vi "Verify powerup.vi"(0 "Measurement Configuration":T3={"Quick Power Down"=FALSE, "Pin Name"=[], "Source Mode"=[], "Start Value"=[], "Target Value"=[], "Compliance Limit"=[], "Sense Mode"=[], "Default Ramp Rate"=[], "Ramp Rate"=[], "Start Delay"=[], "Relative To"=[], "Transient Response"=[], "Data Capture"=FALSE, "Power line frequency"=1} {"Relative To" items=["Power sequence start", "Previous source start", "Previous source end"]; "Power line frequency" items=["50 Hz", "60 Hz"]; "Start Value" format="%#_6p"; "Transient Response" items=["Slow", "Normal", "Fast"]; "Sense Mode" items=["Local Sense", "Remote Sense"]; "Target Value" format="%#_6p"; "Source Mode" items=["DC Voltage", "DC Current"]; "Start Delay" format="%#_6p"; "Compliance Limit" format="%#_6p"; "Ramp Rate" format="%#_6p"}, 5 "Measurements":T1, 11 "error in (no error)":errorcluster) -> (4 "Error[]":string[](array[string]), 15 "error out":errorcluster)   [LabVIEW 2024, in "devicePowerSequencerCoreLogic.lvlib"]
doc: "Checks status of pins to verify the power up"
uses:
  devicePowerSequencerCoreLogic.lvlib
  Measurement Configuration.ctl
  controls/Source Mode.ctl
  controls/Sense Mode.ctl
  controls/Relative To.ctl
  controls/Transient Response.ctl
  controls/Power line frequency.ctl
  controls/Measurements.ctl
  controls/Voltage and Current Measurements.ctl
  <vilib>/Utility/error.llb/Clear Errors.vi
  Form Error Message.vi/4da3fa3f-d6a2-4c6b-9c9c-fc44bca91f7b.vi
  <vilib>/Utility/error.llb/Error Cluster From Error Code.vi
  Device Power Sequencer.lvlib
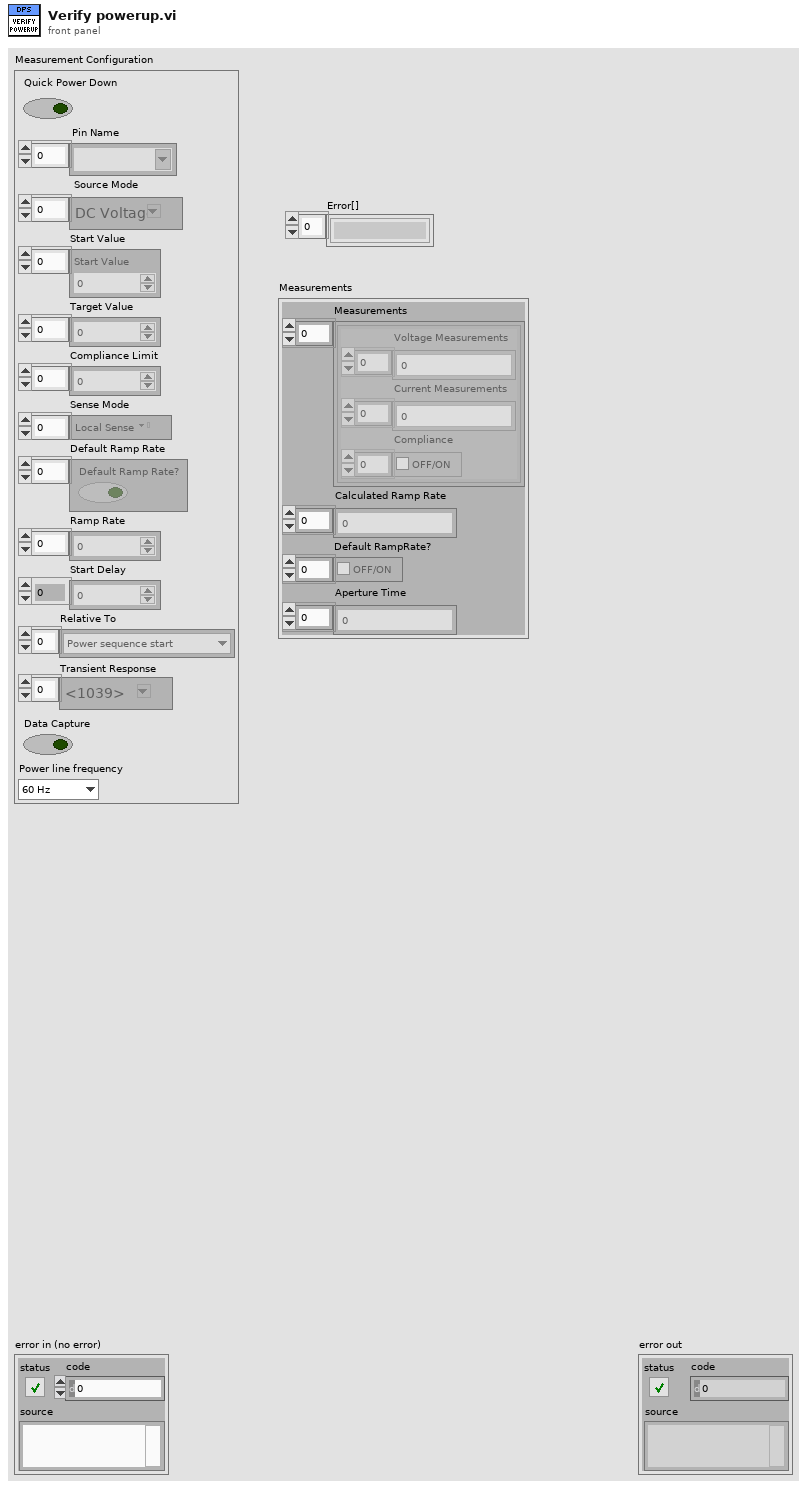
[diagram p1: front panel]
types:
  T1 = typedef "devicePowerSequencerCoreLogic.lvlib/Measurements.ctl" = cluster{"Measurements":T2[], "Calculated Ramp Rate":dbl[], "Default RampRate?":bool[], "Aperture Time":dbl[]}
  T2 = typedef "devicePowerSequencerCoreLogic.lvlib/Voltage and Current Measurements.ctl" = cluster{"Voltage Measurements":dbl[], "Current Measurements":dbl[], "Compliance":bool[]}
  T3 = typedef "Device Power Sequencer.lvlib/Measurement Configuration.ctl" = cluster{"Quick Power Down":bool, "Pin Name":string[], "Source Mode":T4[], "Start Value":dbl[], "Target Value":dbl[], "Compliance Limit":dbl[], "Sense Mode":T5[], "Default Ramp Rate":bool[], "Ramp Rate":dbl[], "Start Delay":dbl[], "Relative To":T6[], "Transient Response":T7[], "Data Capture":bool, "Power line frequency":T8}
  T4 = typedef "Device Power Sequencer.lvlib/Source Mode.ctl" = i32
  T5 = typedef "Device Power Sequencer.lvlib/Sense Mode.ctl" = i32
  T6 = typedef "Device Power Sequencer.lvlib/Relative To.ctl" = u32
  T7 = typedef "Device Power Sequencer.lvlib/Transient Response.ctl" = i32
  T8 = typedef "Device Power Sequencer.lvlib/Power line frequency.ctl" = u32
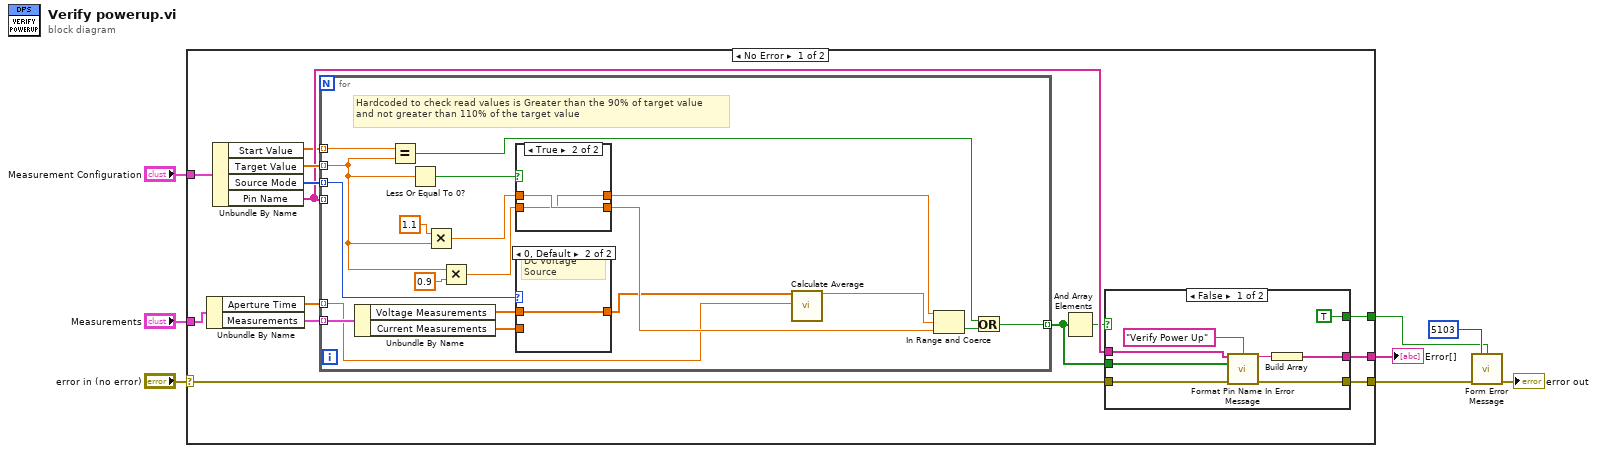
[diagram p0: block diagram]
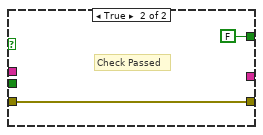
[diagram p2: hidden frame]
diagram:
  n1 = case shown="No Error" "error in (no error)" {
    selector: "error in (no error)" -> [w9 w58]
    tunnel: [w16 w58] -> w4
    tunnel: "Measurement Configuration" -> [w22 _]
    tunnel: "Measurements" -> [w19 _]
    tunnel: [w15 _] -> w2
    tunnel: [w12 _] -> w1
    frame No Error {
      n2 = Unbundle By Name(w19) -> ("Aperture Time"=w10:dbl[], "Measurements"=w18:T2[])
      n3 = Unbundle By Name(w22) -> ("Start Value"=w11:dbl[], "Target Value"=w21:dbl[], "Source Mode"=w20:T4[], "Pin Name"=w17:string[])
      n4 = for {
        tunnel: w18 -> [w51] mode=indexing
        tunnel: w21 -> [w36] mode=indexing
        tunnel: w20 -> [w50] mode=indexing
        tunnel: w17 -> [_] mode=indexing
        tunnel: [w39] -> w13 mode=indexing
        tunnel: w11 -> [w37] mode=indexing
        tunnel: w10 -> [w34] mode=indexing
        # "Hardcoded to check read values is Greater than the 90% of target value\nand not greater than 110% of the target value"
        n5 = Unbundle By Name(w51) -> ("Voltage Measurements"=w47:dbl[], "Current Measurements"=w49:dbl[])
        n6 = Equal?(x=w37, y=w36) -> (x = y?=w38:bool)
        n7 = Less Or Equal To 0?(x=w36) -> (x <= 0?=w41:bool)
        n8 = Multiply(x=1.1, y=w36) -> (x*y=w45:dbl)
        n9 = Multiply(x=w36, y=0.9) -> (x*y=w44:dbl)
        n10 = case shown="True" w41 {
          tunnel: w45 -> [w53 w55]
          tunnel: [w52 w55] -> w43
          tunnel: w44 -> [w52 w54]
          tunnel: [w53 w54] -> w42
          frame False {
          }
          frame True {
          }
        }
        n11 = case shown="0, Default" w50 {
          tunnel: w49 -> [w56 _]
          tunnel: w47 -> [_ w57]
          tunnel: [w56 w57] -> w35
          frame 1 {
            # "DC Current Source"
          }
          frame 0, Default {
            # "DC Voltage Source"
          }
        }
        n12 = call "Calculate Average.vi"("Measurements"=w35, "Aperture Time"=w34) -> ("Average level"=w33:dbl)  [unwired: 13 in]
        n13 = In Range and Coerce(upper limit=w42, x=w33, lower limit=w43) -> (In Range?=w40:bool)  [unwired: 1 out]
        n14 = Or(x=w38, y=w40) -> (x .or. y?=w39:bool)
      }
      n15 = And Array Elements(Boolean array=w13) -> (logical AND=w14:bool)
      n16 = case shown="False" w14 {
        tunnel: w17 -> [w30 _]
        tunnel: [w28 w31] -> w16
        tunnel: [w27 _] -> w15
        tunnel: w13 -> [w26 _]
        tunnel: [TRUE ("Boolean") FALSE ("Boolean")] -> w12
        tunnel: w9 -> [w23 w31]
        frame False {
          n17 = call "Format Pin Name In Error Message.vi"("Pin Name"=w30, "Parameter Name"="Verify Power Up", "Error[]"=w26, "error in"=w23) -> ("Error Message"=w29:string, "error out"=w28:errorcluster)  [unwired: 10 in]
          n18 = Build Array(w29) -> (w27:string[])
        }
        frame True {
          # "Check Passed"
        }
      }
    }
    frame Error {
    }
  }
  "Error[]" <- w2
  n19 = call "Form Error Message.vi"("error code (0)"=5103, "Error?"=w1, "error in (no error)"=w4) -> ("error out"=→"error out":errorcluster)  [unwired: 12 in]
